vi "GetRefPropGen.vi"(0 "Controls":refnum<vi>[](array[refnum]), 1 "Énum":enum16{"Label Text", "Enable"}(ring), 11 "Error in":errorcluster) -> (4 "Controls Out":refnum<vi>[](array[refnum]), 6 "Enable":T1(array[ring]), 8 "LabelText":string[](array[string]), 15 "Error out":errorcluster)   [LabVIEW 2019]
doc: "Ce VI ouvre le fichier de sauvegarde des modèles et lit les positions du modèle spécifié."
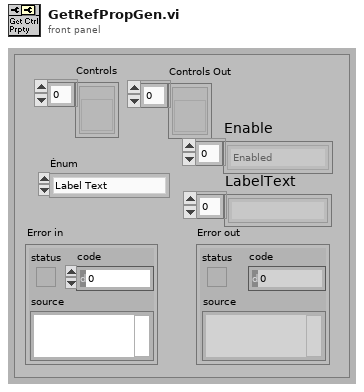
[diagram p1: front panel]
types:
  T1 = enum8{"Enabled", "Disabled", "Disabled and Grayed Out"}[]
  T2 = enum8{"Enabled", "Disabled", "Disabled and Grayed Out"}
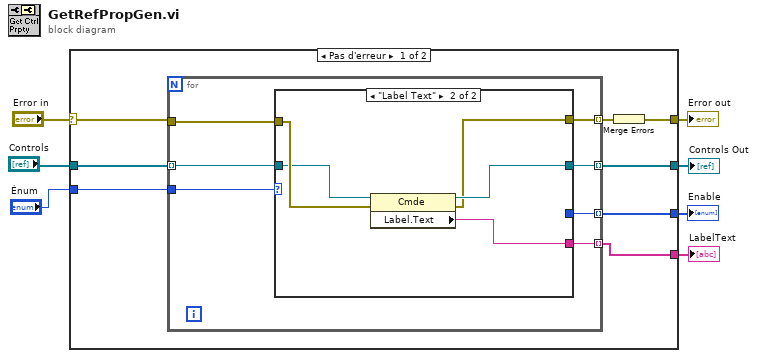
[diagram p0: block diagram]
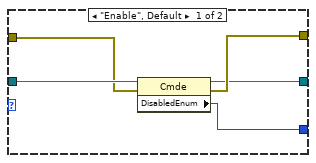
[diagram p2: hidden frame]
diagram:
  n1 = case shown="Pas d'erreur" "Error in" {
    selector: "Error in" -> [w15 w34]
    tunnel: [w13 w34] -> w7
    tunnel: [w12 w33] -> w5
    tunnel: "Controls" -> [w11 w33]
    tunnel: "Énum" -> [w10 _]
    tunnel: [w9 _] -> w2
    tunnel: [w8 _] -> w1
    frame No Error {
      n2 = for {
        tunnel: w11 -> [w22] mode=indexing
        tunnel: w15 -> [w21]
        tunnel: [w20] -> w14 mode=indexing
        tunnel: [w19] -> w12 mode=indexing
        tunnel: w10 -> [w18]
        tunnel: [w17] -> w9 mode=indexing
        tunnel: [w16] -> w8 mode=indexing
        n3 = case shown="\"Label Text\"" w18 {
          tunnel: w22 -> [w27 w31]
          tunnel: w21 -> [w26 w32]
          tunnel: [w25 w29] -> w20
          tunnel: [w24 w30] -> w19
          tunnel: [w23 _] -> w17
          tunnel: [_ w28] -> w16
          frame "Enable", Default {
            n4 = property class="Cmde"(reference=w27, error in=w26) -> (reference out=w24:refnum<vi>, error out=w25:errorcluster, "DisabledEnum"=w23:T2)
          }
          frame "Label Text" {
            n5 = property class="Cmde"(reference=w31, error in=w32) -> (reference out=w30:refnum<vi>, error out=w29:errorcluster, "Label.Text"=w28:string)
          }
        }
      }
      n6 = Merge Errors(w14) -> (w13:errorcluster)
    }
    frame Error {
    }
  }
  "Error out" <- w7
  "Controls Out" <- w5
  "Enable" <- w2
  "LabelText" <- w1
